vi "RectangularROIonMatchPOS (SubVI).vi"(10 "Matches (pixel)":T1(array[cluster]), 11 "ROI Descriptor before matches":T3={"Global Rectangle"=[675, 567, 1751, 1642], "Contours"=[{"ID"=enum."External", "Type"=7, "Coordinates"=[1212, 1104, 85, 537, 0, 0]}]} {"Contours"."Type" items=["No Selection", "Point", "Line", "Rectangle", "Oval", "Polygon", "Freehand Region", "Annulus", "Unused2", "Unused3", "Broken Line", "Freehand Line", "Rotated Rectangle"]}) -> (3 "ROI Descriptor after matches":T2)   [LabVIEW 2016]
panel:
  out "Bounding Box[3]":cluster{"x":sgl, "y":sgl}
  out "Bounding Box[1]":cluster{"x":sgl, "y":sgl}
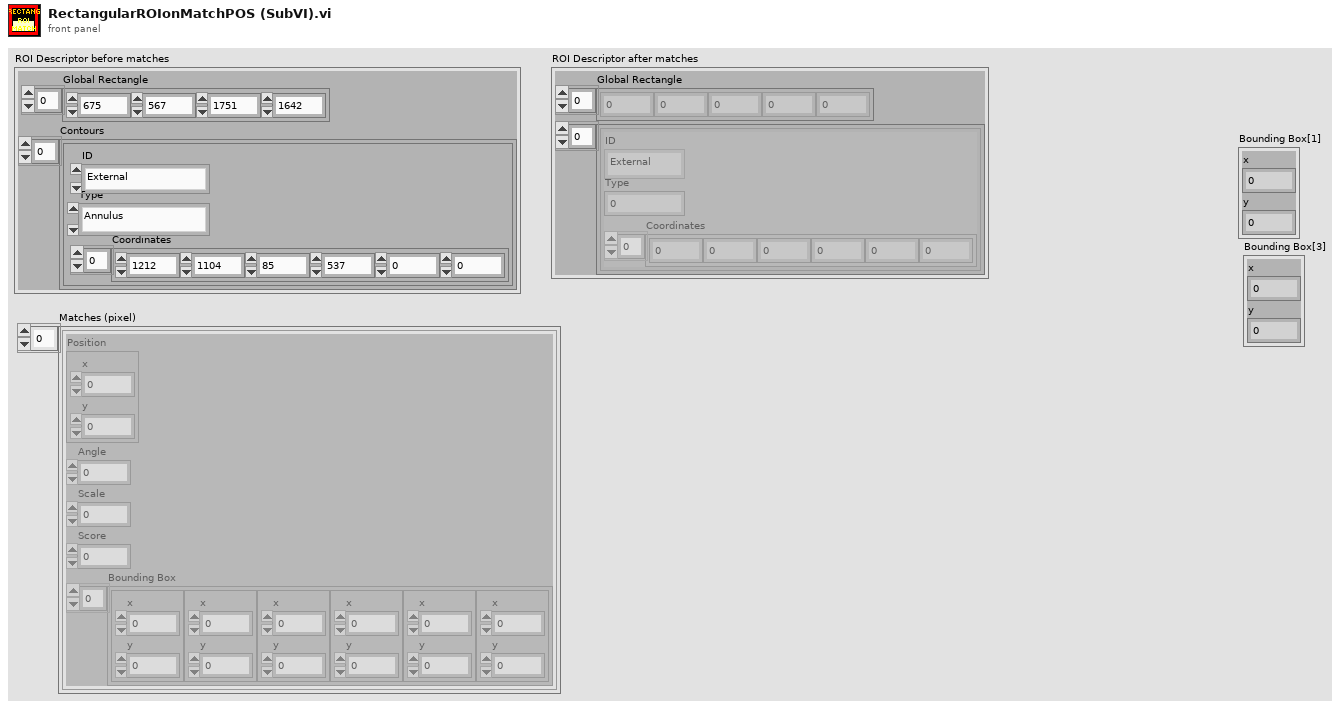
[diagram p1: front panel]
types:
  T1 = cluster{"Position":cluster{"x":sgl, "y":sgl}, "Angle":sgl, "Scale":sgl, "Score":sgl, "Bounding Box":cluster{"x":sgl, "y":sgl}[]}[]
  T2 = cluster{"Global Rectangle":i32[], cluster{"ID":enum32{"External", "Internal"}, "Type":u32, "Coordinates":i32[]}[]}
  T3 = cluster{"Global Rectangle":i32[], "Contours":cluster{"ID":enum32{"External", "Internal"}, "Type":u32, "Coordinates":i32[]}[]}
  T4 = cluster{"ID":enum32{"External", "Internal"}, "Type":u32, "Coordinates":i32[]}[]
  T5 = cluster{"Bounding Box[0]":cluster{"x":sgl, "y":sgl}, "Bounding Box[1]":cluster{"x":sgl, "y":sgl}, "Bounding Box[2]":cluster{"x":sgl, "y":sgl}, "Bounding Box[3]":cluster{"x":sgl, "y":sgl}, "Bounding Box[4]":cluster{"x":sgl, "y":sgl}, "Bounding Box[5]":cluster{"x":sgl, "y":sgl}, "Bounding Box[6]":cluster{"x":sgl, "y":sgl}, "Bounding Box[7]":cluster{"x":sgl, "y":sgl}, "Bounding Box[8]":cluster{"x":sgl, "y":sgl}}
  T6 = cluster{"ID":enum32{"External", "Internal"}, "Type":u32, "Coordinates":i32[]}
  T7 = cluster{"Coordinates":i32[], cluster{"ID":enum32{"External", "Internal"}, "Type":u32, "Coordinates":i32[]}[]}
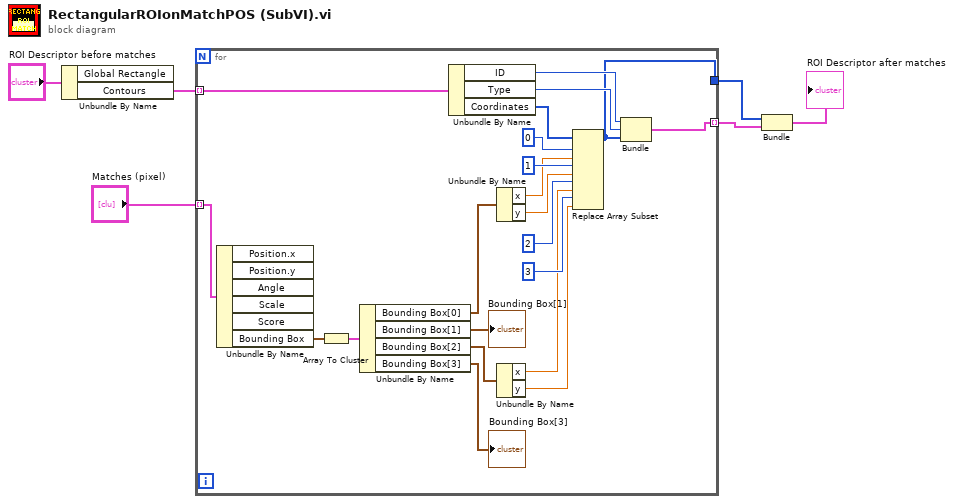
[diagram p0: block diagram]
diagram:
  n1 = Unbundle By Name("ROI Descriptor before matches") -> ("Contours"=w4:T4)  [unwired: 1 out]
  n2 = for {
    tunnel: w4 -> [w27] mode=indexing
    tunnel: "Matches (pixel)" -> [w23] mode=indexing
    tunnel: [w20] -> w6 mode=indexing
    tunnel: [w7] -> w2
    n3 = Unbundle By Name(w23) -> ("Bounding Box"=w19:cluster{"x":sgl, "y":sgl}[])  [unwired: 5 out]
    n4 = Array To Cluster(array=w19) -> (cluster=w18:T5)
    n5 = Unbundle By Name(w18) -> ("Bounding Box[0]"=w15:cluster{"x":sgl, "y":sgl}, "Bounding Box[1]"=→"Bounding Box[1]":cluster{"x":sgl, "y":sgl}, "Bounding Box[2]"=w10:cluster{"x":sgl, "y":sgl}, "Bounding Box[3]"=→"Bounding Box[3]":cluster{"x":sgl, "y":sgl})
    n6 = Unbundle By Name(w27) -> ("ID"=w21:enum32{"External", "Internal"}, "Type"=w22:u32, "Coordinates"=w26:i32[])
    n7 = Unbundle By Name(w15) -> ("x"=w14:sgl, "y"=w13:sgl)
    n8 = Unbundle By Name(w10) -> ("x"=w9:sgl, "y"=w8:sgl)
    n9 = Replace Array Subset(array=w26, new element #1=w14, index #1=0 ("index"), new element #2=w13, index #2=1 ("index"), new element #3=w9, index #3=2 ("index"), new element #4=w8, index #4=3 ("index")) -> (w7:i32[])
    n10 = Bundle("ID"=w21, "Type"=w22, "Coordinates"=w7) -> (w20:T6)  [unwired: 1 in]
  }
  n11 = Bundle("Coordinates"=w2, w6) -> (→"ROI Descriptor after matches":T7)  [unwired: 1 in]
